vi "Read Locale.vi"(11 "MsgSerializer":refnum<class "MsgSerializer.JSON.lvclass">) -> (2 "Locale":string, 3 "MsgSerializer":refnum<class "MsgSerializer.JSON.lvclass">)   [LabVIEW 2020]
uses:
  MsgSerializer/MsgSerializer.JSON.lvclass
  C:/projects/caraya/src/classes/MsgSerializer/MsgSerializer.lvclass
  C:/projects/caraya/src/classes/MsgSerializer.JSON/MsgSerializer/MsgSerializer.JSON.lvclass
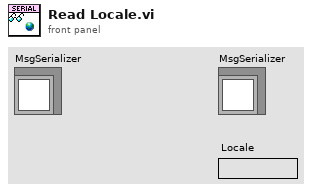
[diagram p1: front panel]
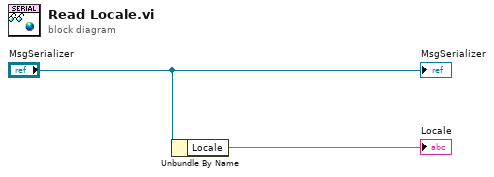
[diagram p0: block diagram]
diagram:
  n1 = Unbundle By Name("MsgSerializer") -> ("Locale"=→"Locale")
  "MsgSerializer" <- "MsgSerializer"
